vi "G#Debugger_Close.vi"(0 "refs":T1, 5 "error in (no error)":errorcluster) -> (19 "error out":errorcluster)   [LabVIEW 2020, in "G#Debugger.lvlib"]
uses:
  <vilib>/addons/_AddQ/G#Debugger/G#Debugger.lvlib
  <vilib>/addons/_AddQ/G#Debugger/private/G#Debugger_Refs.ctl
  <vilib>/addons/_AddQ/G#Object/utils/G#Object_ClassInfoType.ctl
  <vilib>/addons/_AddQ/G#Object/G#Object.lvclass
  <vilib>/addons/_AddQ/G#Object/utils/G#Object_ObjectInfoType.ctl
  <vilib>/addons/_AddQ/G#Object/utils/G#Object_CreateMethod.ctl
  <vilib>/addons/_AddQ/G#Debugger/private/G#Debugger_SubPanelInfo.ctl
  <vilib>/addons/_AddQ/G#Object/utils/G#Object_ClassHierarchy.ctl
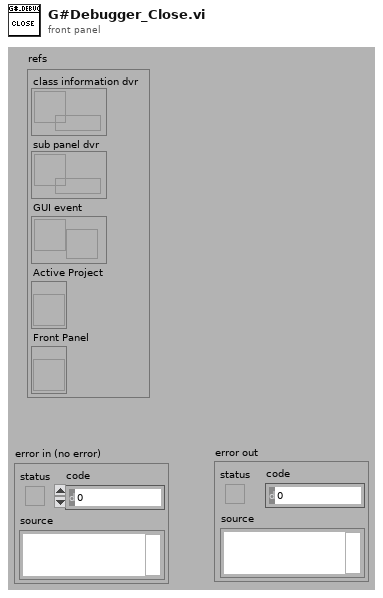
[diagram p1: front panel]
types:
  T1 = typedef "G#Debugger.lvlib/G#Debugger_Refs.ctl" = cluster{"class information dvr":refnum<data-value>, "sub panel dvr":refnum<data-value>, "GUI event":refnum<user-event>, "Active Project":refnum<vi>, "Front Panel":refnum<vi>}
  T2 = typedef "G#Debugger.lvlib/G#Debugger_SubPanelInfo.ctl" = cluster{"Ref":refnum<class "G#Object.lvclass">, "class hierarchy":T3[], "class attributes":path[], "object attributes":path[], "inheritance index":i32, "is class attributes":bool, "vi reference":refnum<vi>}
  T3 = typedef "G#Object.lvclass/G#Object_ClassHierarchy.ctl" = cluster{"ClassName":string, "FullClassName":string, "ClassPath":path, "IsLeaf":bool}
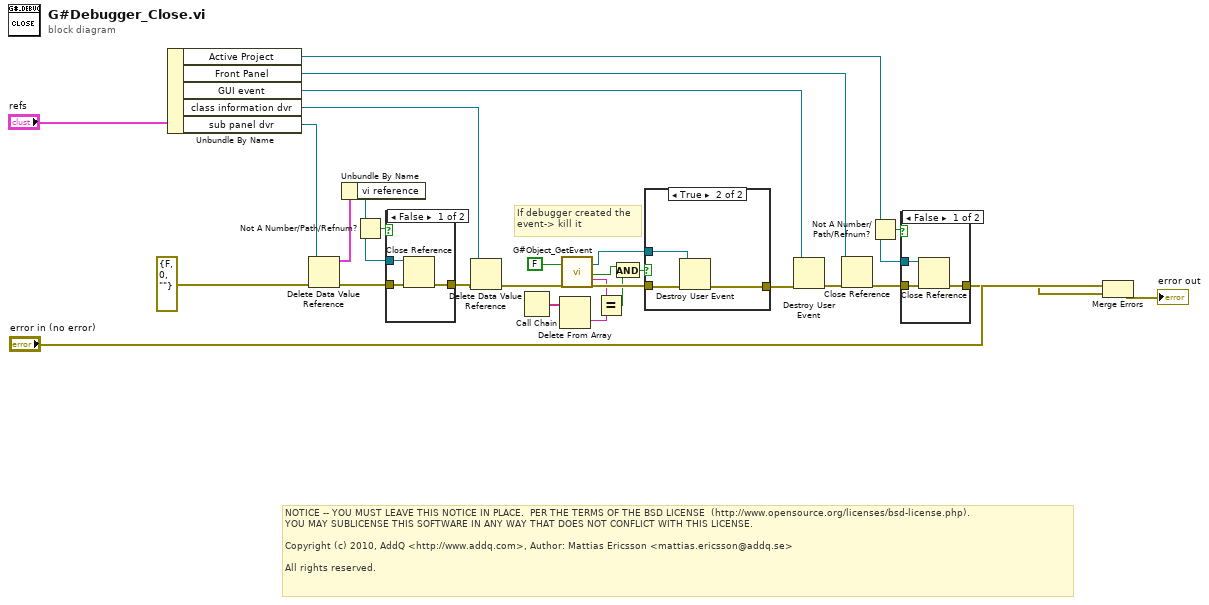
[diagram p0: block diagram]
diagram:
  # "If debugger created the\nevent-> kill it"
  # "NOTICE -- YOU MUST LEAVE THIS NOTICE IN PLACE.  PER THE TERMS OF THE BSD LICENSE  (http://www.opensource.org/licenses/bsd-license.php).\nYOU MAY SUBLICENSE THIS SOFTWARE IN ANY WAY THAT DOES NOT CONFLICT WITH THIS LICENSE.\n\nCopyright (c) 2010, AddQ <http://www.addq.com>, Author: Mattias Ericsson <mattias.ericsson@addq.se>\n\nAll rights reserved."
  n1 = Unbundle By Name("refs") -> ("Active Project"=w11:refnum<vi>, "Front Panel"=w2:refnum<vi>, "GUI event"=w19:refnum<user-event>, "class information dvr"=w22:refnum<data-value>, "sub panel dvr"=w23:refnum<data-value>)
  n2 = Delete Data Value Reference(data value reference=w23, error in=errorcluster {"status"=FALSE, "code"=0, "source"=""} ("error in (no error)")) -> (data value=w28:T2, error out=w27:errorcluster)
  n3 = Unbundle By Name(w28) -> ("vi reference"=w24:refnum<vi>)
  n4 = Not A Number/Path/Refnum?(number/path/refnum=w24) -> (NaN/Path/Refnum?=w26:bool)
  n5 = case shown="False" w26 {
    tunnel: w27 -> [w32 w33]
    tunnel: [w31 w33] -> w25
    tunnel: w24 -> [w30 _]
    frame False {
      n6 = Close Reference(reference=w30, error in (no error)=w32) -> (error out=w31:errorcluster)
    }
    frame True {
    }
  }
  n7 = Delete Data Value Reference(data value reference=w22, error in=w25) -> (error out=w18:errorcluster)  [unwired: 1 out]
  n8 = Call Chain() -> (call chain=w9:string[])
  n9 = Delete From Array(array=w9) -> (deleted portion=w8:string)  [unwired: 2 in, 1 out]
  n10 = call <vilib>:"G#Object_GetEvent.vi"("create if needed (T)"=FALSE ("create if needed"), "error in (no error)"=w18) -> ("G# event"=w14:refnum<user-event>, "valid"=w6:bool, "event owner"=w7:string, "error out"=w16:errorcluster)  [unwired: 13 in, 1 out]
  n11 = Equal?(x=w7, y=w8) -> (x = y?=w5:bool)
  n12 = And(x=w6, y=w5) -> (x .and. y?=w15:bool)
  n13 = case shown="True" w15 {
    tunnel: w16 -> [w34 w37]
    tunnel: w14 -> [_ w36]
    tunnel: [w34 w35] -> w13
    frame False {
    }
    frame True {
      n14 = Destroy User Event(user event=w36, error in=w37) -> (error out=w35:errorcluster)
    }
  }
  n15 = Destroy User Event(user event=w19, error in=w13) -> (error out=w4:errorcluster)
  n16 = Close Reference(reference=w2, error in (no error)=w4) -> (error out=w3:errorcluster)
  n17 = Not A Number/Path/Refnum?(number/path/refnum=w11) -> (NaN/Path/Refnum?=w12:bool)
  n18 = case shown="False" w12 {
    tunnel: w3 -> [w40 w41]
    tunnel: [w39 w41] -> w10
    tunnel: w11 -> [w38 _]
    frame False {
      n19 = Close Reference(reference=w38, error in (no error)=w40) -> (error out=w39:errorcluster)
    }
    frame True {
    }
  }
  n20 = Merge Errors("error in (no error)", w10) -> (→"error out":errorcluster)
